vi "Nidaq_6009.vi"() -> ()   [LabVIEW 2011]
doc: "E-Mail Notification.vi demonstrates a temperature analysis application and how to send a message under certain Limit and Acquistion conditions. This VI asks for recipients for e-mail messages and a valid mail server; reads a simulated temperature; alarms if it is outside a given range;and sends an e-mail referencing condition to listed recipients.\n\nThe Mail Server must be valid for the example to work properly."
uses:
  <vilib>/Analysis/NI_AALPro.lvlib
panel:
  in  "a":dbl=115.08
  in  "b":dbl=2.8238
  out "number of samples":dbl
  out "mean":dbl
  out "min":dbl
  out "max":dbl
  out "standard deviation":dbl
  in  "dt":dbl=1.0 format="%0.2f"
  out "dX/dt":dbl[](array[numeric])
  out "Histogram":dynamicdata(graph)
  out "Time has Elapsed":bool
  in  "tempeartura":dbl
  out "Temperatura":dynamicdata(graph)
  in  "OHL":bool
  in  "High Limit":dbl(knob)=85.0 scale=70.0..300.0 scale format="%0.0f"
  in  "Low Limit":dbl(knob)=80.07649936341923 scale=0.0..300.0 scale format="%0.0f"
  out "OHL Display":bool
  out "Thermometer":dbl(slide)=79.58984375 scale=70.0..90.0 scale format="%0.2f"
  in  "Acquisition":bool=TRUE
  in  "Update Period":dbl(slide)=1.0 scale=0.0..2.0 scale format="%0.2f"
  out "Temp History":T1(graph)
  # "Temperature History"
  # "System Controls"
  # "Current Temperature"
  # "(deg F)"
  # "(s)"
  # "on\noff"
  # "Temperature Range"
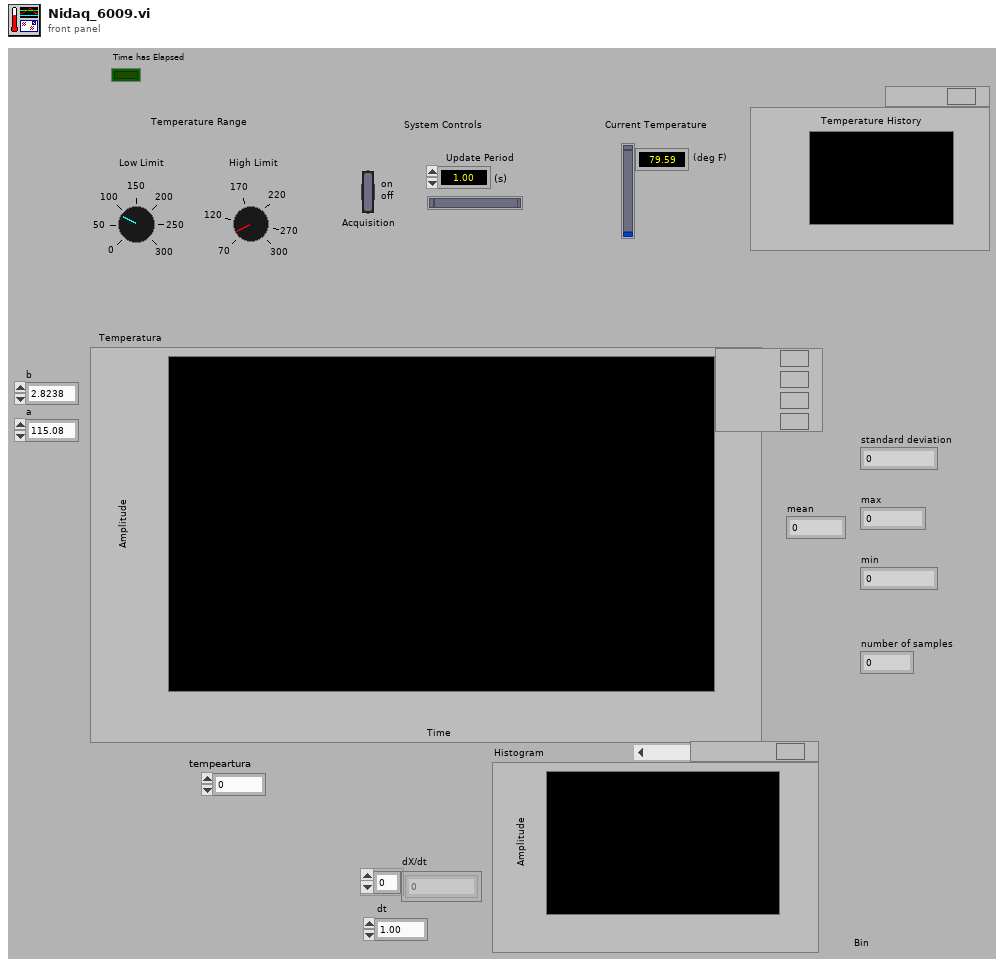
[diagram p1: front panel]
types:
  T1 = cluster{"Temperature":dbl, "High Limit":dbl, "Low Limit":dbl}
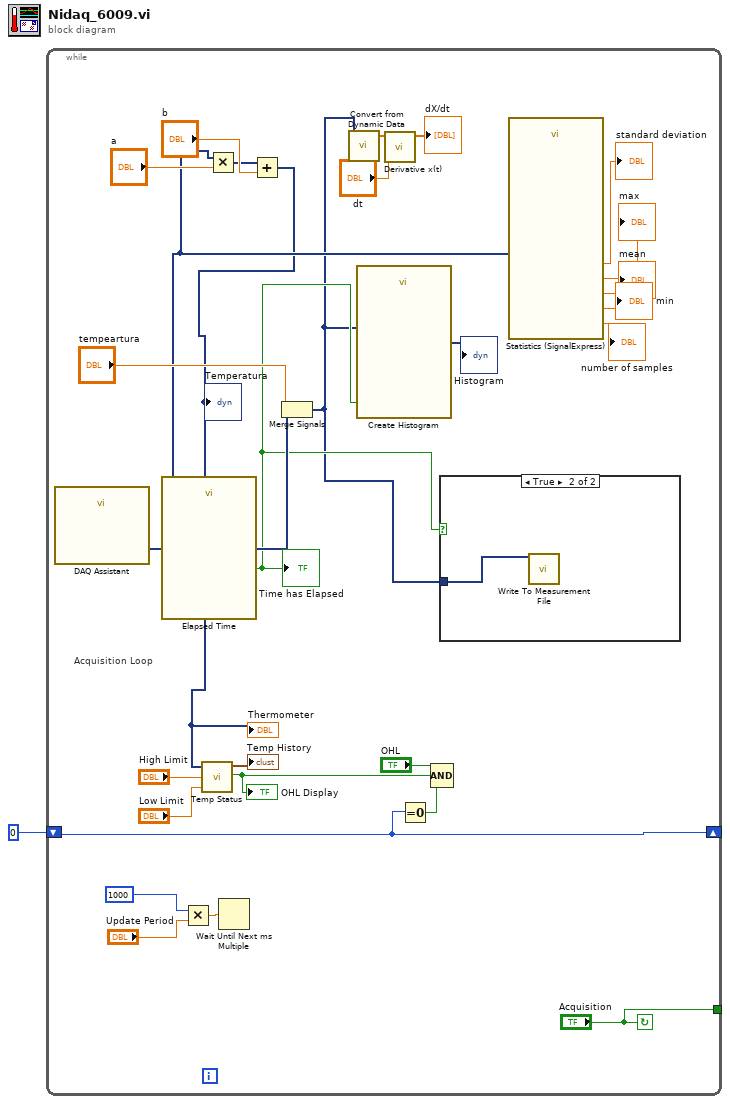
[diagram p0: block diagram]
diagram:
  # "Acquisition Loop"
  n1 = while {
    shift-left: 0 -> [w2]
    shift-right: [w2] -> _
    tunnel: ["Acquisition"] -> _
    stop <- "Acquisition" continue-if-true
    n2 = call "DAQ Assistant"() -> ("data"=w16:dynamicdata)  [unwired: 17 in, 2 out]
    n3 = call "Elapsed Time"() -> ("Time has Elapsed"=w9:bool)  [unwired: 12 in, 7 out]
    "Time has Elapsed" <- w9
    n4 = Multiply(x=1000, y="Update Period") -> (x*y=w22:dbl)
    n5 = Multiply(x=w16, y="a") -> (x*y=w15:dynamicdata)
    n6 = Wait Until Next ms Multiple(millisecond multiple=w22) -> ()  [unwired: 1 out]
    n7 = Add(x=w15, y="b") -> (x+y=w3:dynamicdata)
    "Thermometer" <- w3
    "Temperatura" <- w3
    n8 = call "Temp Status.vi"("Low Limit"="Low Limit", "High Limit"="High Limit", "Temperature"=w3) -> ("Over Limit"=w27:bool, "Chart Output"=→"Temp History":T1)  [unwired: 1 out]
    "OHL Display" <- w27
    n9 = Merge Signals("tempeartura", w16) -> (w8:dynamicdata)
    n10 = call "Convert from Dynamic Data"("Dynamic Data Type"=w8) -> ("Array"=w5:dbl[])  [unwired: 3 in]
    n11 = call "Create Histogram"("Reset"=w9, "Signal"=w8) -> ("Histogram"=→"Histogram":dynamicdata)  [unwired: 8 in, 1 out]
    n12 = call <vilib>:"Derivative x(t).vi"("dt"="dt", "X"=w5) -> ("dX/dt"=→"dX/dt":dbl[])  [unwired: 8 in, 1 out]
    n13 = Equal To 0?(x=w2) -> (x = 0?=w26:bool)
    n14 = Compound Arithmetic op=AND("OHL", w27, w26) -> ()  [unwired: 1 out]
    n15 = case shown="True" w9 {
      tunnel: w8 -> [_ w30]
      frame False {
      }
      frame True {
        n16 = call "Write To Measurement File"("Signals"=w30) -> ()  [unwired: 16 in, 3 out]
      }
    }
    n17 = call "Statistics (SignalExpress)"("input signal"=w16) -> ("standard deviation"=→"standard deviation":dbl, "max"=→"max":dbl, "min"=→"min":dbl, "mean"=→"mean":dbl, "number of samples"=→"number of samples":dbl)  [unwired: 12 in, 2 out]
  }
